vi "MT Add AWGN.vi"(0 "input complex waveform":T1={"t0"=0.0, "dt"=1.0, "Y"=[]} {"Y" format="%.3f"; "dt" format="%^.2e"; "t0" format="%.4f"}, 5 "samples per symbol (16)":i32=16, 7 "bits per symbol (1)":i32=1, 9 "Eb/N0 (10 dB)":dbl=10.0 format="%.2f", 11 "error in (no error)":errorcluster, 12 "seed in (0xFFFFFFFF)":i32=-1 format="%.0x", 13 "reset? (T)":bool=TRUE) -> (4 "output complex waveform":T1 {"Y" format="%.3f"; "dt" format="%^.2e"; "t0" format="%.4f"}, 10 "seed out":i32 format="%.0x", 15 "error out":errorcluster)   [LabVIEW 2020, in "niDMT.lvlib"]
doc: "Generates zero-mean complex additive white Gaussian noise (AWGN) with uniform power spectral density and adds it to the complex baseband modulated waveform."
uses:
  <vilib>/addons/Modulation/niDMT.lvlib
  <vilib>/addons/Modulation/Analog/controls/Complex Data Waveform.ctl
  <vilib>/addons/Modulation/Digital/Support/Common/Validators/mod_Validate Samples Per Symbol.vi
  <vilib>/addons/Modulation/Analog/support/Validators/mod_Validate Complex Waveform.vi
  <vilib>/addons/Modulation/Analog/support/Validators/mod_WFErrorHandler.vi
  <vilib>/addons/Modulation/Digital/General/subVIs/mod_Generate Bits PN Sequence.vi
  <vilib>/addons/Modulation/niAMT.lvlib
  <vilib>/Analysis/NI_AALBase.lvlib
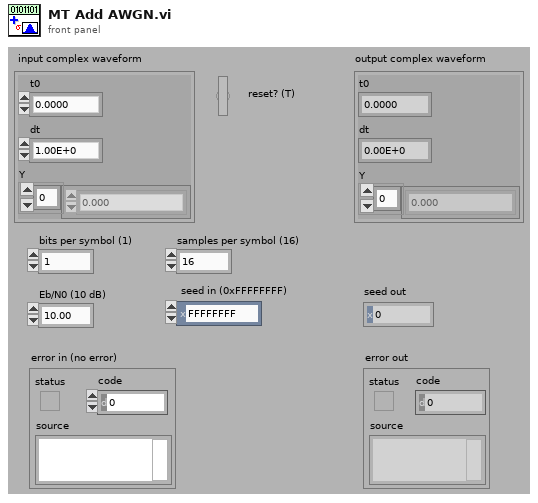
[diagram p1: front panel]
types:
  T1 = typedef "niAMT.lvlib/Complex Data Waveform.ctl" = cluster{"t0":dbl, "dt":dbl, "Y":cdb[]}
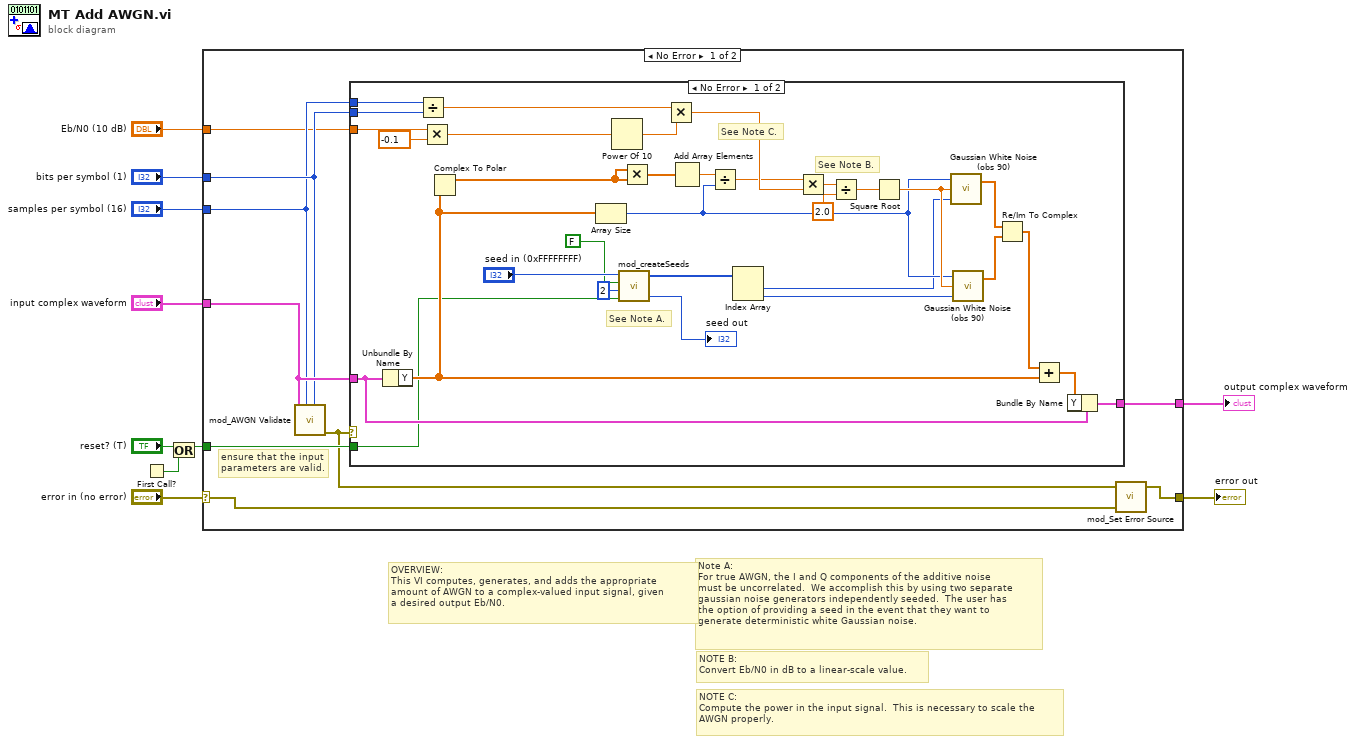
[diagram p0: block diagram]
diagram:
  # "NOTE C:\nCompute the power in the input signal.  This is necessary to scale the\nAWGN properly."
  # "NOTE B:\nConvert Eb/N0 in dB to a linear-scale value."
  # "OVERVIEW:\nThis VI computes, generates, and adds the appropriate\namount of AWGN to a complex-valued input signal, given\na desired output Eb/N0."
  # "Note A:\nFor true AWGN, the I and Q components of the additive noise\nmust be uncorrelated.  We accomplish this by using two separate\ngaussian noise generators independently seeded.  The user has\nthe option of providing a seed in the event that they want to\ngenerate deterministic white Gaussian noise."
  n1 = First Call?() -> (First Call?: T/F=w1:bool)
  n2 = Or(x="reset? (T)", y=w1) -> (x .or. y?=w2:bool)
  n3 = case shown="No Error" "error in (no error)" {
    selector: "error in (no error)" -> [w11 w53]
    tunnel: "input complex waveform" -> [w19 _]
    tunnel: "bits per symbol (1)" -> [w17 _]
    tunnel: "samples per symbol (16)" -> [w16 _]
    tunnel: w2 -> [w18 _]
    tunnel: "Eb/N0 (10 dB)" -> [w15 _]
    tunnel: [w14 _] -> w5
    tunnel: [w13 w53] -> w4
    frame No Error {
      # "ensure that the input parameters are valid."
      n4 = call <vilib>:"mod_AWGN Validate.vi"("Bits Per Symbol (1)"=w17, "Samples Per Symbol (16)"=w16, "Input Complex Waveform"=w19) -> ("error out"=w12:errorcluster)  [unwired: 1 in, 7 out]
      n5 = case shown="No Error" w12 {
        tunnel: w19 -> [w32 w52]
        tunnel: w18 -> [w26 _]
        tunnel: w17 -> [w40 _]
        tunnel: w16 -> [w39 _]
        tunnel: w15 -> [w37 _]
        tunnel: [w30 w52] -> w14
        frame No Error {
          # "See Note A."
          # "See Note B."
          # "See Note C."
          n6 = Unbundle By Name(w32) -> ("Y"=w33:cdb[])
          n7 = Divide(x=w39, y=w40) -> (x/y=w42:dbl)
          n8 = Multiply(x=w37, y=-0.1) -> (x*y=w36:dbl)
          n9 = Complex To Polar(r * e^(i*theta)=w33) -> (r=w29:dbl[])  [unwired: 1 out]
          n10 = Array Size(array=w33) -> (size(s)=w45:i32)
          n11 = Power Of 10(x=w36) -> (10^x=w35:dbl)
          n12 = call <vilib>:"mod_createSeeds.vi"("Reset? (T)"=w26, "# of seeds to create"=2, "Allow Neg if not already? (T)"=FALSE, "seed in (0xFFFFFFFF)"="seed in (0xFFFFFFFF)") -> ("Next seed"=→"seed out":i32, "Seeds"=w24:i32[])  [unwired: 1 out]
          n13 = Multiply(x=w29, y=w29) -> (x*y=w28:dbl[])
          n14 = Multiply(x=w42, y=w35) -> (x*y=w43:dbl)
          n15 = Add Array Elements(numeric array=w28) -> (sum=w41:dbl)
          n16 = Divide(x=w41, y=w45) -> (x/y=w34:dbl)
          n17 = Index Array(array=w24) -> (element #1=w22:i32, element #2=w23:i32)  [unwired: 2 in]
          n18 = Multiply(x=w34, y=w43) -> (x*y=w51:dbl)
          n19 = Divide(x=w51, y=2.0) -> (x/y=w49:dbl)
          n20 = Square Root(x=w49) -> (sqrt(x)=w48:dbl)
          n21 = call <vilib>:"Gaussian White Noise (obs 90).vi"("seed"=w22, "standard deviation"=w48, "samples"=w45) -> ("Gaussian noise pattern"=w46:dbl[])  [unwired: 1 out]
          n22 = call <vilib>:"Gaussian White Noise (obs 90).vi"("seed"=w23, "standard deviation"=w48, "samples"=w45) -> ("Gaussian noise pattern"=w47:dbl[])  [unwired: 1 out]
          n23 = Re/Im To Complex(1:w47, 2:w46) -> (0:w50:cdb[])
          n24 = Add(x=w50, y=w33) -> (x+y=w31:cdb[])
          n25 = Bundle By Name(cluster=w32, "Y"=w31) -> (w30:T1)
        }
        frame Error {
        }
      }
      n26 = call <vilib>:"mod_Set Error Source.vi"("initial error in (no error)"=w11, "final error in (no error)"=w12) -> ("error out"=w13:errorcluster)  [unwired: 1 in, 2 out]
    }
    frame Error {
    }
  }
  "error out" <- w4
  "output complex waveform" <- w5
